vi "PicoScope Read.vi"(2 "WFD-Ref Ch-B":refnum<vi>, 3 "WFD-Ref Ch-A":refnum<vi>, 4 "Acquisition Settings":T4={"preTriggerSamples"=0, "postTriggerSamples"=1000, "timebase"=62500, "Down-Sample Mode"=0, "Down Sample Ratio"=1, "Oversample"=0} {"Down Sample Ratio" min=1 step=1; "Down-Sample Mode" items=["None"=0, "Aggregate"=1, "Decimate"=2, "Average"=4]; "postTriggerSamples" max=10000 step=100}, 5 "Trigger Settings":T5={"Trigger Enabled"=TRUE, "Trigger Source"=enum."Channel A", "Trigger Threshold (Volts)"=0.0, "Trigger Direction"=2, "Trigger Delay (samples)"=0, "Auto Trigger Time (ms)"=1000} {"Trigger Direction" items=["Rising"=2, "Falling"=3]}, 6 "Channel B Settings":T2={"Enabled"=TRUE, "Coupling"=1, "Range"=8, "Analogue Offset"=0.0} {"Range" items=["20 mV"=1, "50 mV"=2, "100 mV"=3, "200 mV"=4, "500 mV"=5, "1 V"=6, "2 V"=7, "5 V"=8, "10 V"=9, "20 V"=10]; "Coupling" items=["AC", "DC"]}, 7 "Channel A Settings":T2={"Enabled"=TRUE, "Coupling"=1, "Range"=7, "Analogue Offset"=0.0} {"Range" items=["20 mV"=1, "50 mV"=2, "100 mV"=3, "200 mV"=4, "500 mV"=5, "1 V"=6, "2 V"=7, "5 V"=8, "10 V"=9, "20 V"=10]; "Coupling" items=["AC", "DC"]}, 8 "error in":errorcluster, 9 "Max Adc value":i16, 10 "Device Info":T1, 11 "handle":i16) -> (0 "error out":errorcluster)   [LabVIEW 2018]
panel:
  out "Channel B":cluster{i32, "Sample Internal":sgl, dbl[]}(graph)
  out "Properties Panel":T3 {"Max Total Capture Time Available (sec)" format="%.3p"; "Sample Frequency" format="%.3p"; "Sample Internal" format="%.3p"; "Max Samples Available" format="%.3p"; "Total Capture Time (sec)" format="%.3p"}
  out "Channel A":cluster{i32, "Sample Internal":sgl, dbl[]}(graph)
  # "127"
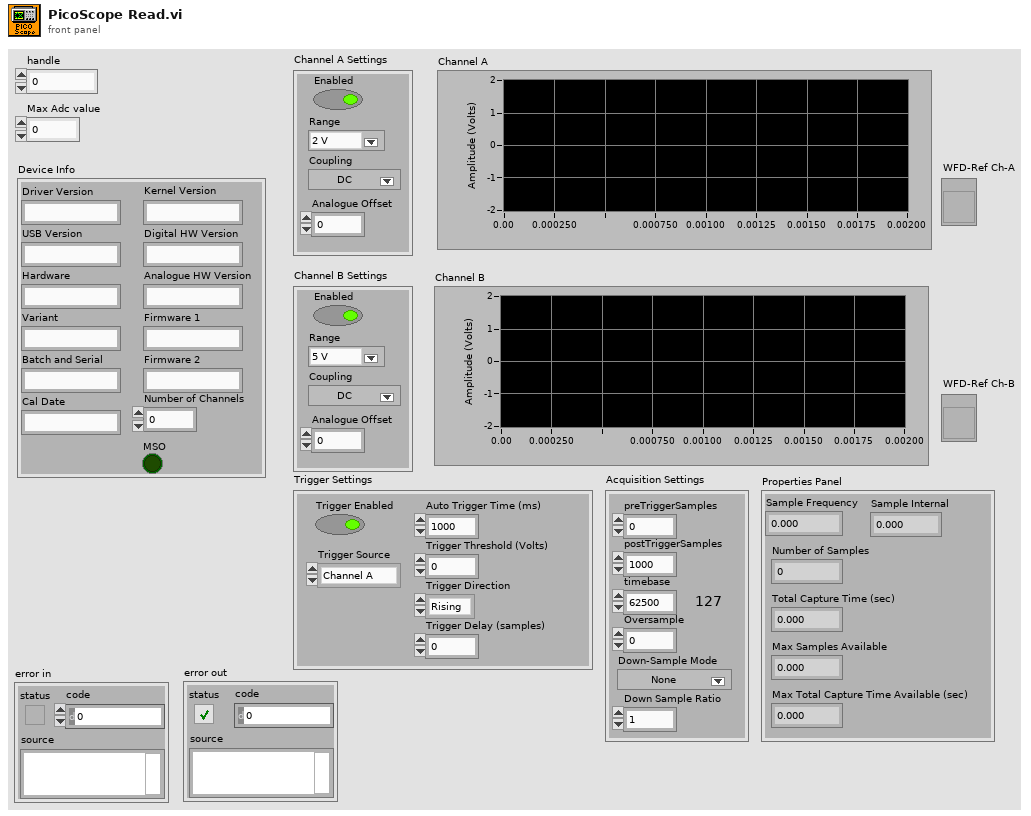
[diagram p1: front panel]
types:
  T1 = cluster{"Driver Version":string, "USB Version":string, "Hardware":string, "Variant":string, "Batch and Serial":string, "Cal Date":string, "Kernel Version":string, "Digital HW Version":string, "Analogue HW Version":string, "Firmware 1":string, "Firmware 2":string, "MSO":bool, "Number of Channels":i16}
  T2 = cluster{"Enabled":bool, "Coupling":i16, "Range":u16, "Analogue Offset":sgl}
  T3 = cluster{"Sample Frequency":sgl, "Sample Internal":sgl, "Max Samples Available":i32, "Number of Samples":u32, "Total Capture Time (sec) ":sgl, "Max Total Capture Time Available (sec)":sgl}
  T4 = cluster{"preTriggerSamples":u32, "postTriggerSamples":u32, "timebase":u32, "Down-Sample Mode":i32, "Down Sample Ratio":u32, "Oversample":i16}
  T5 = cluster{"Trigger Enabled":bool, "Trigger Source":enum16{"Channel A", "Channel B", "Channel C", "Channel D", "Ext."}, "Trigger Threshold (Volts)":dbl, "Trigger Direction":u16, "Trigger Delay (samples)":u32, "Auto Trigger Time (ms)":i16}
  T6 = cluster{"Channel D Buffer":i16[], "Channel C Buffer":i16[], "Channel B Buffer":i16[], "Channel A Buffer":i16[], "Port 0  Buffer ":i16[], "Port 1 Buffer ":i16[]}
  T7 = cluster{i32, "Sample Internal":sgl, "Data (Volts)":dbl[]}
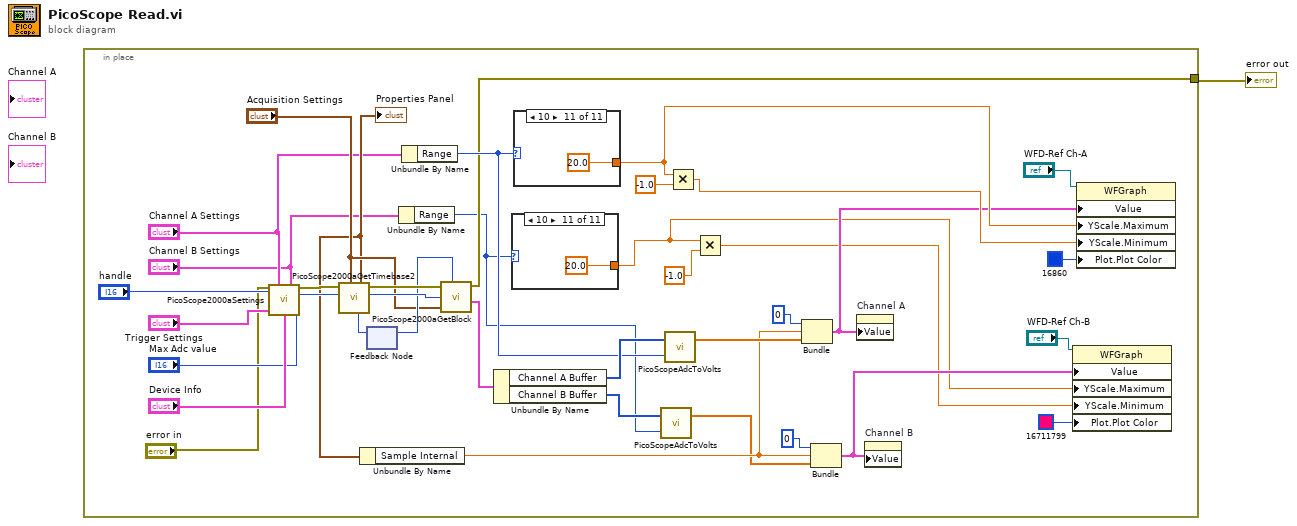
[diagram p0: block diagram]
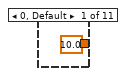
[diagram p2: hidden frame]
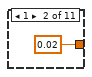
[diagram p3: hidden frame]
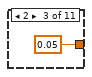
[diagram p4: hidden frame]
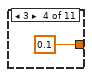
[diagram p5: hidden frame]
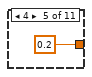
[diagram p6: hidden frame]
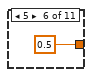
[diagram p7: hidden frame]
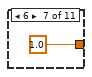
[diagram p8: hidden frame]
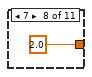
[diagram p9: hidden frame]
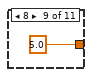
[diagram p10: hidden frame]
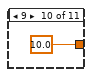
[diagram p11: hidden frame]
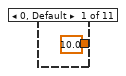
[diagram p12: hidden frame]
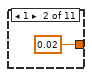
[diagram p13: hidden frame]
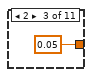
[diagram p14: hidden frame]
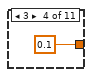
[diagram p15: hidden frame]
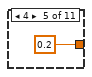
[diagram p16: hidden frame]
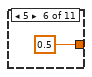
[diagram p17: hidden frame]
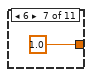
[diagram p18: hidden frame]
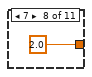
[diagram p19: hidden frame]
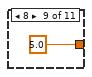
[diagram p20: hidden frame]
diagram:
  n1 = in-place {
    in-place-border: [w14] -> w1
    n2 = call "PicoScope2000aSettings.vi"("error in"="error in", "Channel A Settings"="Channel A Settings", "Channel B Settings"="Channel B Settings", "handle in"="handle", "Trigger Settings"="Trigger Settings", "Device Info"="Device Info", "Max_adc"="Max Adc value") -> ("error out"=w38:errorcluster, "handle out"=w37:i16)  [unwired: 6 in, 1 out]
    n3 = feedback #1() -> (w33:u32)  [unwired: 1 in]
    n4 = call "PicoScope2000aGetTimebase2.vi"("Number of Samples"=w33, "Acquisition Settings"="Acquisition Settings", "handle in"=w37, "error in (no error)"=w38) -> ("handle out"=w35:i16, "error out"=w36:errorcluster, "Properties Panel"=w29:T3)  [unwired: 5 in]
    "Properties Panel" <- w29
    n5 = Unbundle By Name(w29) -> ("Sample Internal"=w21:sgl)
    n6 = Unbundle By Name("Channel B Settings") -> ("Range"=w5:u16)
    n7 = Unbundle By Name("Channel A Settings") -> ("Range"=w23:u16)
    n8 = call "PicoScope2000aGetBlock.vi"("error in"=w36, "handle in"=w35, "Acquisition Settings"="Acquisition Settings") -> ("noOfSamples"=w34:u32, "error out"=w14:errorcluster, "Buffers (Max or non-aggregated)"=w31:T6)  [unwired: 2 in, 3 out]
    n9 = feedback-in #1(w34) -> ()
    n10 = Unbundle By Name(w31) -> ("Channel A Buffer"=w28:i16[], "Channel B Buffer"=w24:i16[])
    n11 = case shown="10" w5 {
      tunnel: [10.0 0.02 0.05 0.1 0.2 0.5 1.0 2.0 5.0 10.0 20.0] -> w3
      frame 0, Default {
      }
      frame 1 {
      }
      frame 2 {
      }
      frame 3 {
      }
      frame 4 {
      }
      frame 5 {
      }
      frame 6 {
      }
      frame 7 {
      }
      frame 8 {
      }
      frame 9 {
      }
      frame 10 {
      }
    }
    n12 = case shown="10" w23 {
      tunnel: [10.0 0.02 0.05 0.1 0.2 0.5 1.0 2.0 5.0 10.0 20.0] -> w16
      frame 0, Default {
      }
      frame 1 {
      }
      frame 2 {
      }
      frame 3 {
      }
      frame 4 {
      }
      frame 5 {
      }
      frame 6 {
      }
      frame 7 {
      }
      frame 8 {
      }
      frame 9 {
      }
      frame 10 {
      }
    }
    n13 = call "PicoScopeAdcToVolts.vi"("Range Index"=w5, "Data"=w24) -> ("Data (Volts)"=w20:dbl[])  [unwired: 1 in]
    n14 = call "PicoScopeAdcToVolts.vi"("Range Index"=w23, "Data"=w28) -> ("Data (Volts)"=w26:dbl[])  [unwired: 1 in]
    n15 = Multiply(x=w16, y=-1.0) -> (x*y=w15:dbl)
    n16 = Multiply(x=w3, y=-1.0) -> (x*y=w2:dbl)
    n17 = Bundle(0, "Sample Internal"=w21, "Data (Volts)"=w26) -> (w13:T7)  [unwired: 1 in]
    n18 = Bundle(0, "Sample Internal"=w21, "Data (Volts)"=w20) -> (w18:T7)  [unwired: 1 in]
    n19 = property on="Channel A" class="WFGraph (strict)"("Value"=w13) -> ()  [unwired: 2 in, 2 out]
    n20 = property on="Channel B" class="WFGraph (strict)"("Value"=w18) -> ()  [unwired: 2 in, 2 out]
    n21 = property class="WFGraph"(reference="WFD-Ref Ch-B", "Value"=w18, "YScale.Maximum"=w3, "YScale.Minimum"=w2, "Plot.Plot Color"=u32 16711799) -> ()  [unwired: 1 in, 2 out]
    n22 = property class="WFGraph"(reference="WFD-Ref Ch-A", "Value"=w13, "YScale.Maximum"=w16, "YScale.Minimum"=w15, "Plot.Plot Color"=u32 16860) -> ()  [unwired: 1 in, 2 out]
  }
  "error out" <- w1
